vi "HART_init.vi"(8 "error in":errorcluster, 11 "resource name":refnum<visa-resource-name>) -> (0 "error out":errorcluster)   [LabVIEW 2016]
uses:
  <vilib>/Instr/_visa.llb/VISA Configure Serial Port (Instr).vi
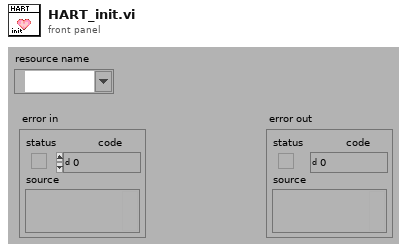
[diagram p1: front panel]
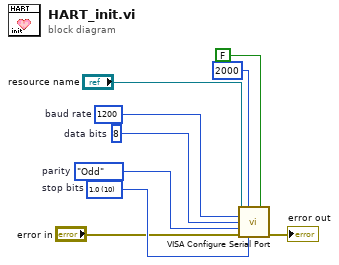
[diagram p0: block diagram]
diagram:
  w5 = u16 10 items=["1.0"=10, "1.5"=15, "2.0"=20]  # stop bits
  w6 = enum16{"None", "Odd", "Even", "Mark", "Space"}."Odd"  # parity
  w7 = u16 8  # data bits
  w8 = u32 1200  # baud rate
  n1 = call-poly "VISA Configure Serial Port"("VISA resource name"="resource name", "timeout (10sec)"=u32 2000, "Enable Termination\nChar (T)"=FALSE ("Enable Termination\nChar (T)"), "baud rate (9600)"=w8, "data bits (8)"=w7, "parity (0:none)"=w6, "error in (no error)"="error in", "stop bits (10: 1 bit)"=w5) -> ("error out"=→"error out":errorcluster)  [unwired: 6 in, 1 out]
